vi "Example 03 - Lua Functions.vi"() -> ()   [LabVIEW 2020]
uses:
  Lua for LabVIEW/Lua/Lua.lvclass
panel:
  in  "lua script":string="-- define a function\nfunction my_func(x, y)\n  return 2 * (x + y)\nend"
  in  "y":dbl=2.75 format="%#_13g"
  in  "x":dbl=1.25 format="%#_13g"
  out "error out":errorcluster
  out "result":dbl
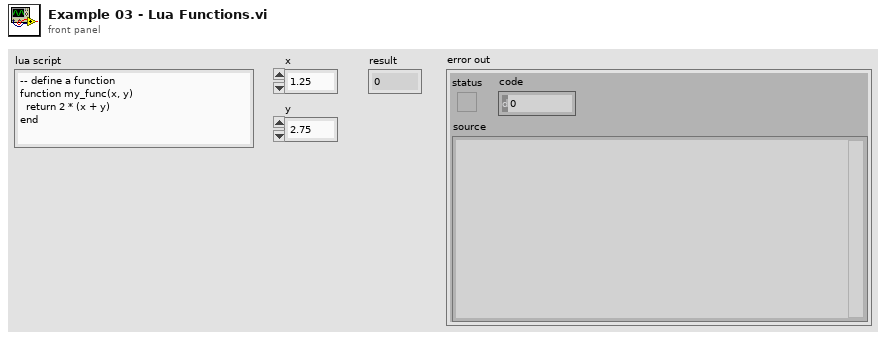
[diagram p1: front panel]
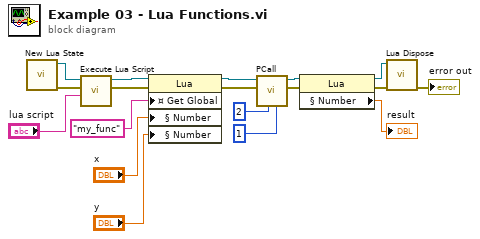
[diagram p0: block diagram]
diagram:
  n1 = call "New Lua State.vi"() -> ("error out"=w5:errorcluster, "Lua out"=w18:refnum<class "Lua.lvclass">)  [unwired: 10 in]
  n2 = call-dynamic "Execute Lua Script.vi"("lua script"="lua script", "error in (no error)"=w5, "Lua in"=w18) -> ("error out"=w3:errorcluster, "Lua out"=w17:refnum<class "Lua.lvclass">)  [unwired: 7 in]
  n3 = property class="Lua"(reference=w17, error in=w3, "¤ Get Global"="my_func" ("(State) Get Global"), "§ Number"="x", "§ Number"="y") -> (reference out=w13:refnum<class "Lua.lvclass">, error out=w2:errorcluster)
  n4 = call-dynamic "PCall.vi"("nresults"=1, "nargs"=2, "error in (no error)"=w2, "Lua in"=w13) -> ("error out"=w1:errorcluster, "Lua out"=w10:refnum<class "Lua.lvclass">)  [unwired: 6 in]
  n5 = property class="Lua"(reference=w10, error in=w1) -> (reference out=w8:refnum<class "Lua.lvclass">, error out=w7:errorcluster, "§ Number"=→"result":dbl)
  n6 = call-dynamic "Lua Dispose.vi"("error in (no error)"=w7, "Lua in"=w8) -> ("error out"=→"error out":errorcluster)  [unwired: 9 in]
